vi "CAN Signals Monitoring Timing.vi"() -> ()   [LabVIEW 2010]
uses:
  <vilib>/Platform/storage/lvStorage.llb/xStorage/Open Data Storage/Open Data Storage.xnode
  <vilib>/Platform/storage/lvStorage.llb/_openFunction.ctl
  <vilib>/Platform/storage/lvStorage.llb/xStorage/Set Properties/Set Properties.xnode
  <vilib>/Platform/storage/lvStorage.llb/xStorage/Write Data/Write Data.xnode
  <vilib>/Platform/storage/Storage.llb/usiOverwriteOptions.ctl
  <vilib>/Platform/storage/Storage.llb/usiSequenceRepresentation.ctl
  <vilib>/Platform/storage/lvStorage.llb/xStorage/Close Data Storage/Close Data Storage.xnode
  <instrlib>/Tektronix DPO MSO 2000 4000 Series/Public/Data/Read (Single Waveform).vi
  <vilib>/Platform/storage/lvStorage.llb/_openStorageWithRootAutoDetect.vi
  <vilib>/Platform/storage/lvStorage.llb/xStorage/xStorageSupp/ErrorOut.vi
  <vilib>/Platform/storage/Storage.llb/__savePropString.vi
  <vilib>/Platform/storage/Storage.llb/__savePropTime.vi
  <vilib>/Platform/storage/Storage.llb/_createExplicitChildObject.vi
  <vilib>/Platform/storage/lvStorage.llb/_prepDDT.vi
  <vilib>/Platform/storage/lvStorage.llb/_getChannelNameFromDDT.vi
  <vilib>/Platform/storage/lvStorage.llb/_saveDDT.vi
  <vilib>/Platform/storage/Storage.llb/Get Object Info.vi
  <vilib>/Platform/storage/Storage.llb/__closeStorageFromObject.vi
  <instrlib>/Tektronix DPO MSO 2000 4000 Series/Tektronix DPO MSO 2000 4000 Series.lvlib
panel:
  out "String":string
  in  "Select port":string(combo)
  out "Period":dbl
  out "CAN+TIMB":waveform(dbl)(graph)
  in  "Assembled by":string="Alexis Ibarra"
  in  "ABM-S/N":string
  in  "Port":u16(ring) items=["AMB 1", "AMB 2", "AMB 3", "AMB 4", "AMB 5", "AMB 18"]
  in  "Channel A (0: Channel 1)":u16(ring) items=["Channel 1", "Channel 2", "Channel 3", "Channel 4", "Math", "Reference 1", "Reference 2", "Reference 3", "Reference 4"]
  in  "Channel B (1: Channel 2)":u16(ring)=1 items=["Channel 1", "Channel 2", "Channel 3", "Channel 4", "Math", "Reference 1", "Reference 2", "Reference 3", "Reference 4"]
  in  "Maximum Time (10000ms)":u32=20000
  out "CAN":waveform(dbl)(graph)
  out "TIMB":waveform(dbl)(graph)
  in  "DPO-4034 IP Adress":string
  out "error out":errorcluster
  # "Actually ip address\n10.195.18.178"
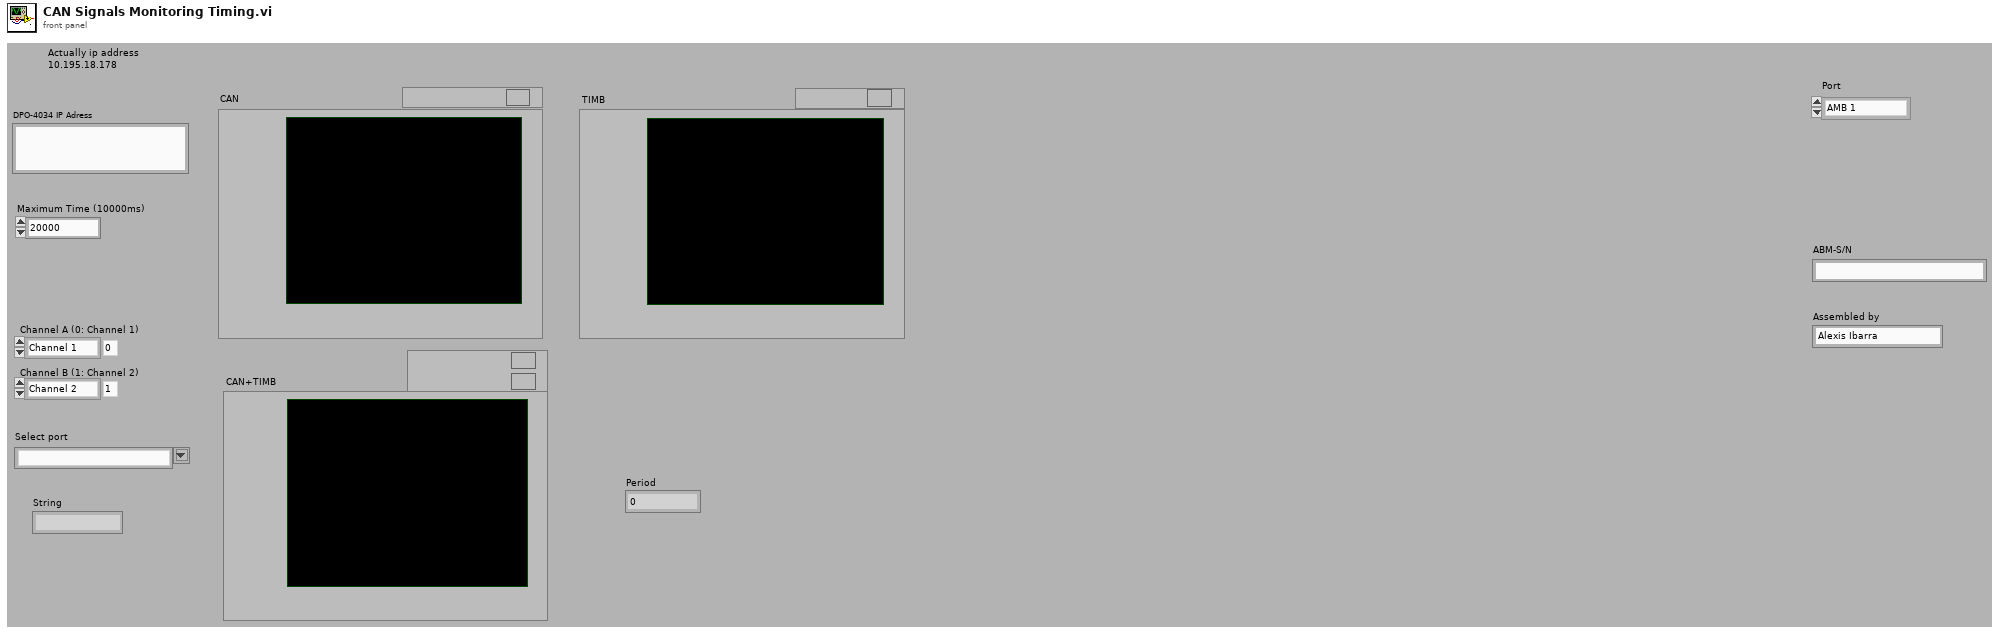
[diagram p1: front panel]
types:
  T1 = enum16{"UPDATE", "READ", "QUERY", "CREATE CHILD", "CREATE", "CONNECT", "DISCONNECT"}
  T2 = typedef "usiOverwriteOptions.ctl" = enum16{"Append values", "Replace values at index", "Replace all values", "Append if timeline aligns"}
  T3 = typedef "usiSequenceRepresentation.ctl" = enum16{"explicit", "implicit"}
  T4 = typedef "_openFunction.ctl" = enum16{"open", "open or create", "create or replace", "create", "open (read only)"}
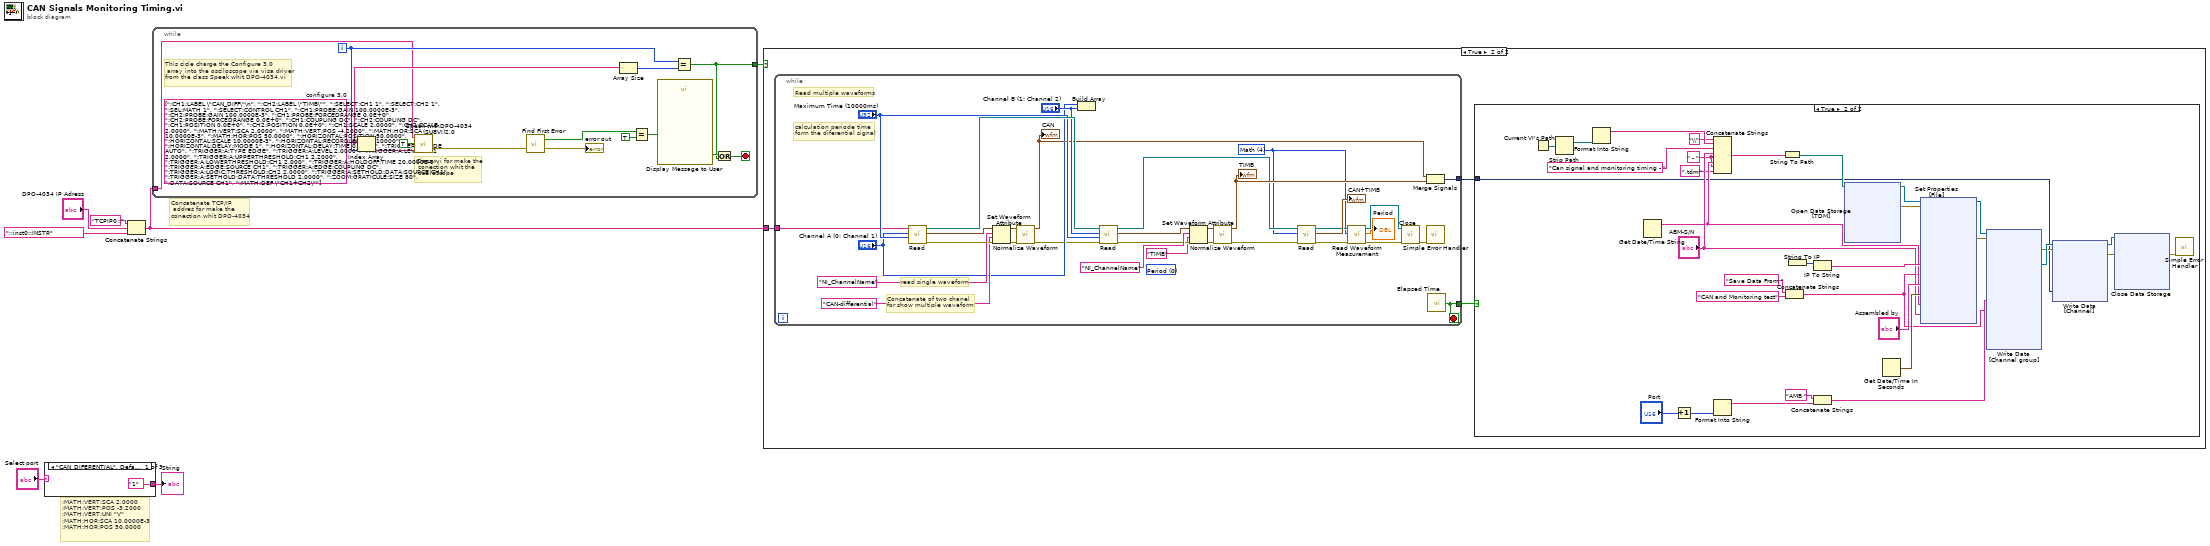
[diagram p0: block diagram]
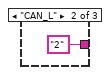
[diagram p2: hidden frame]
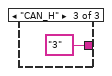
[diagram p3: hidden frame]
diagram:
  # ":MATH:VERT:SCA 2.0000\n:MATH:VERT:POS -3.2000\n:MATH:VERT:UNI \"V\"\n:MATH:HOR:SCA 10.0000E-3\n:MATH:HOR:POS 50.0000"
  # "Concatenate TCP/IP\n addres for make the \nconection whit DPO-4034"
  n1 = case shown="\"CAN_DIFERENTIAL\", Default" "Select port" {
    tunnel: ["1" "2" "3"] -> w1
    frame "CAN_DIFERENTIAL", Default {
    }
    frame "CAN_L" {
    }
    frame "CAN_H" {
    }
  }
  "String" <- w1
  n2 = Concatenate Strings("TCPIP0::", "DPO-4034 IP Adress", "::inst0::INSTR") -> (w3:string)
  n3 = while {
    tunnel: w3 -> [w14]
    tunnel: [w11] -> w4
    i -> [w23]
    stop <- w12 stop-if-true
    w18 = string[] [":CH1:LABEL \"CAN_DIFF\"\n", ":CH2:LABEL \"TIMB\"", ":SELECT:CH1 1", ":SELECT:CH2 1", ":SEL:MATH 1", ":SELECT:CONTROL CH1", ":CH1:PROBE:GAIN 100.0000E-3", ":CH2:PROBE:GAIN 100.0000E-3", ":CH1:PROBE:FORCEDRANGE 0.0E+0", ":CH2:PROBE:FORCEDRANGE 0.0E+0", ":CH1:COUPLING DC", ":CH2:COUPLING DC", ":CH1:POSITION 0.0E+0", ":CH2:POSITION 0.0E+0", ":CH1:SCALE 2.0000", ":CH2:SCALE 2.0000", ":MATH:VERT:SCA 2.0000", ":MATH:VERT:POS -4.2000", ":MATH:HOR:SCA 10.0000E-3", ":MATH:HOR:POS 50.0000", ":HORIZONTAL:POSITION 50.0000", ":HORIZONTAL:SCALE 10.0000E-3", ":HORIZONTAL:RECORDLENGTH 10000", ":HORIZONTAL:DELAY:MODE 1", ":HORIZONTAL:DELAY:TIME 0.0E+0", ":TRIGGER:A:MODE AUTO", ":TRIGGER:A:TYPE EDGE", ":TRIGGER:A:LEVEL 2.0000", ":TRIGGER:A:LEVEL:CH1 2.0000", ":TRIGGER:A:UPPERTHRESHOLD:CH1 2.2000", ":TRIGGER:A:LOWERTHRESHOLD:CH1 2.000", ":TRIGGER:A:HOLDOFF:TIME 20.0000E-9", ":TRIGGER:A:EDGE:SOURCE CH1", ":TRIGGER:A:EDGE:COUPLING DC", ":TRIGGER:A:LOGIC:THRESHOLD:CH2 2.0000", ":TRIGGER:A:SETHOLD:DATA:SOURCE CH1", ":TRIGGER:A:SETHOLD:DATA:THRESHOLD 2.0000", ":ZOOM:GRATICULE:SIZE 80", ":DATA:SOURCE CH1", ":MATH:DEF \"CH1+CH2\""]  # configure 3.0
    # "Class .vi for make the\n conection whit the\n osciloscope"
    # "This cicle charge the Configure 3.0\n array into the osciloscope via visa driver \nfrom the class Speek whit DPO-4034.vi"
    n4 = Index Array "Index Array"(array=w18, index=w23) -> (element=w24:string)
    n5 = call "Speak withDPO-4034 (SUBVI)2.0.vi"("Send Command"=w24, "Send:  TRUE\nRecive: FALSE"=TRUE, "VISA Resource Name"=w14) -> ("error out"=w20:errorcluster)  [unwired: 1 out]
    n6 = call <vilib>:"Find First Error.vi"("error in (no error)"=w20) -> ("error out"=→"error out":errorcluster, "error?"=w15:bool)  [unwired: 3 in]
    n7 = Array Size(array=w18) -> (size(s)=w22:i32)
    n8 = Equal?(x=w15, y=TRUE) -> (x = y?=w17:bool)
    n9 = call "Display Message to User"("Enable"=w17) -> ("OK"=w13:bool)  [unwired: 9 in, 1 out]
    n10 = Equal?(x=w23, y=w22) -> (x = y?=w11:bool)
    n11 = Or(x=w13, y=w11) -> (x .or. y?=w12:bool)
  }
  n12 = case shown="True" w4 {
    tunnel: w3 -> [_ w27]
    frame False {
    }
    frame True {
      n13 = while {
        tunnel: w27 -> [w182]
        tunnel: [w169] -> w26
        tunnel: [w179] -> w25
        stop <- w179 stop-if-true
        (unwired) 0 items=["Period", "Frequency", "Delay", "Rise Time", "Fall Time", "Positive Duty Cycle", "Negative Duty Cycle", "Positive Pulse Width", "Negative Pulse Width", "Burst Width", "Phase", "Positive Overshoot", "Negative Overshoot", "Vpp", "Amplitude", "Voltage High", "Voltage Low", "Voltage Max", "Voltage Min", "Voltage Mean", "Voltage Mean (cycle)", "Voltage RMS", "Voltage RMS (cycle)", "Area", "Cycle Area", "Positive Edge Count", "Negative Edge Count", "Positive Pulse Count", "Negative Pulse Count"] ("Measurement Function (0: Period)")
        w164 = u16 4 items=["Channel 1", "Channel 2", "Channel 3", "Channel 4", "Math", "Reference 1", "Reference 2", "Reference 3", "Reference 4"] ("Channel (0: Channel 1)")
        # "read single waveform"
        # "Concatenate of two chanel \nfor show multiple waveform"
        # "calculation periode time\nform the diferential signal"
        # "Read multiple waveforms"
        n14 = call-poly <instrlib>:"Read.vi"("Maximum Time (10000ms)"="Maximum Time (10000ms)", "Channel (0: Channel 1)"="Channel A (0: Channel 1)", "VISA resource name"=w182) -> ("error out"=w188:errorcluster, "Waveform Graph"=w173:waveform(dbl), "VISA resource name out"=w190:refnum<visa-resource-name>)  [unwired: 6 in]
        n15 = Set Waveform Attribute(4:w188, 5:"CAN-differential" ("name"), 6:"NI_ChannelName" ("name"), 7:w173) -> (0:w176:errorcluster, 3:w178:waveform(dbl))  [unwired: 1 out]
        n16 = call <vilib>:"Normalize Waveform.vi"("error in (no error)"=w176, "waveform in"=w178) -> ("error out"=w175:errorcluster, "normalized waveform"=w171:waveform(dbl))  [unwired: 6 in, 2 out]
        "CAN" <- w171
        n17 = Build Array("Channel A (0: Channel 1)", "Channel B (1: Channel 2)") -> ()  [unwired: 1 out]
        n18 = call-poly <instrlib>:"Read.vi"("error in (no error)"=w175, "Maximum Time (10000ms)"="Maximum Time (10000ms)", "Channel (0: Channel 1)"="Channel B (1: Channel 2)", "VISA resource name"=w190) -> ("error out"=w185:errorcluster, "Waveform Graph"=w172:waveform(dbl), "VISA resource name out"=w167:refnum<visa-resource-name>)  [unwired: 5 in]
        n19 = Set Waveform Attribute(4:w185, 5:"TIMB" ("name"), 6:"NI_ChannelName" ("name"), 7:w172) -> (0:w174:errorcluster, 3:w177:waveform(dbl))  [unwired: 1 out]
        n20 = call <vilib>:"Normalize Waveform.vi"("error in (no error)"=w174, "waveform in"=w177) -> ("error out"=w168:errorcluster, "normalized waveform"=w170:waveform(dbl))  [unwired: 6 in, 2 out]
        "TIMB" <- w170
        n21 = call-poly <instrlib>:"Read.vi"("error in (no error)"=w168, "Channel (0: Channel 1)"=w164, "VISA resource name"=w167) -> ("error out"=w163:errorcluster, "Waveform Graph"=→"CAN+TIMB":waveform(dbl), "VISA resource name out"=w165:refnum<visa-resource-name>)  [unwired: 6 in]
        n22 = call <instrlib>:"Read Waveform Measurement.vi"("error in (no error)"=w163, "Channel (0: Channel 1)"=w164, "VISA resource name"=w165) -> ("error out"=w161:errorcluster, "Measurement Value"=→"Period":dbl, "VISA resource name out"=w162:refnum<visa-resource-name>)  [unwired: 6 in]
        n23 = call <instrlib>:"Close.vi"("error in (no error)"=w161, "VISA resource name"=w162) -> ("error out"=w191:errorcluster)  [unwired: 9 in]
        n24 = Merge Signals(w171, w170) -> (w169:dynamicdata)
        n25 = call <vilib>:"Simple Error Handler.vi"("error in (no error)"=w191) -> ()  [unwired: 4 in, 5 out]
        n26 = call "Elapsed Time"() -> ("Time has Elapsed"=w179:bool)  [unwired: 12 in, 7 out]
      }
      n27 = case shown="True" w25 {
        tunnel: w26 -> [_ w28]
        frame False {
        }
        frame True {
          w40 = " - " ("string")
          n28 = Current VI's Path() -> (path=w54:path)
          n29 = Strip Path(path=w54) -> (stripped path=w55:path)  [unwired: 1 out]
          n30 = Format Into String "Format Into String"(w55) -> (resulting string=w53:string)  [unwired: 3 in, 1 out]
          n31 = Get Date/Time String() -> (date string=w41:string)  [unwired: 3 in, 1 out]
          n32 = Increment(x="Port") -> (x+1=w29:u16)
          n33 = Concatenate Strings "Concatenate Strings"(w53, "\\", "Can signal and monitoring timing - " ("string"), "ABM-S/N", w40, w41, w40, ".tdm") -> (w57:string)
          n34 = Format Into String "Format Into String"(w29) -> (resulting string=w37:string)  [unwired: 3 in, 1 out]
          n35 = String To Path(string=w57) -> (path=w58:path)
          n36 = Concatenate Strings "Concatenate Strings"("Save Data From ", "CAN and Monitoring test") -> (w31:string)
          n37 = String To IP() -> (0:w47:u32)  [unwired: 1 in]
          n38 = IP To String(2:w47) -> (0:w48:string)  [unwired: 1 in]
          n39 = Concatenate Strings "Concatenate Strings"("AMB ", w37) -> (w34:string)
          n40 = xnode "Open Data Storage\n[TDM]"("file path"=w58) -> ("storage refnum (file)"=w51:refnum<k20>, "error out"=w38:errorcluster)  [unwired: 4 in, 1 out]
          n41 = Get Date/Time In Seconds() -> (seconds since 1Jan1904=w52:timestamp)
          n42 = xnode "Set Properties\n[File]"("Name"=w48, "Description"=w31, "Author"="Assembled by", "Time stamp"=w52, "Date"=w41, "ABM_SerialNumber"="ABM-S/N", "storage refnum (file)"=w51, "error in"=w38) -> ("storage refnum (file) out"=w36:refnum<k20>, "error out"=w35:errorcluster)
          n43 = xnode "Write Data\n[Channel group]"("Name"=w34, "Description"=w31, "storage refnum (file)"=w36, "error in"=w35) -> ("error out"=w32:errorcluster, "storage refnum (channel group)"=w33:refnum<k20>)  [unwired: 3 in, 1 out]
          n44 = xnode "Write Data\n[Channel]"("Signal"=w28, "storage refnum (channel group)"=w33, "error in"=w32) -> ("storage refnum (channel group) out"=w45:refnum<k20>, "error out"=w44:errorcluster)  [unwired: 2 in, 1 out]
          n45 = xnode "Close Data Storage\n"("storage refnum (channel group)"=w45, "error in (no error)"=w44) -> ("error out"=w46:errorcluster)  [unwired: 1 out]
          n46 = call <vilib>:"Simple Error Handler.vi"("error in (no error)"=w46) -> ()  [unwired: 1 in, 8 out]
        }
      }
    }
  }
